vi "Measure.vi"(8 "error in (no error)":errorcluster, 11 "Instruments in":refnum<class "Instruments.lvclass">) -> (0 "error out":errorcluster, 3 "Instruments out":refnum<class "Instruments.lvclass">)   [LabVIEW 2023, in "Instruments.lvlib" / "Instruments.lvclass"]
doc: "<b>Measure</b>\nMust be overridden by descendent classes.\nCall parent method must be called <b>after</b> the override\n\n<b>Instrument </b> layer reads the measured private data, and enqueues the data for logging\n\nImmediate Descendants of the measure routine should override the measure routine by implementing class specific override methods. The immediate descendant is the only class that should override measure, and their descendants should provide an application speceific method for acquiring data. \n\nThis approach guarantees a common reporting method for instrument telemetry regardless of the specific device used."
uses:
  Library/Instruments.lvclass
  Library/Instruments.lvclass/Instruments.ctl
  builds/Framework/Engine.lvlibp/Engine/Accessors/Read Report Q.vi
  builds/Framework/Actor Framework.lvlibp/1abvi3w/vi.lib/ActorFramework/Actor/Read Actor Label.vi
  builds/Tools/QDMH.lvlibp/Private/Enqueue Single Element.vi
  builds/Tools/QDMH.lvlibp/Library/QDMH.lvclass
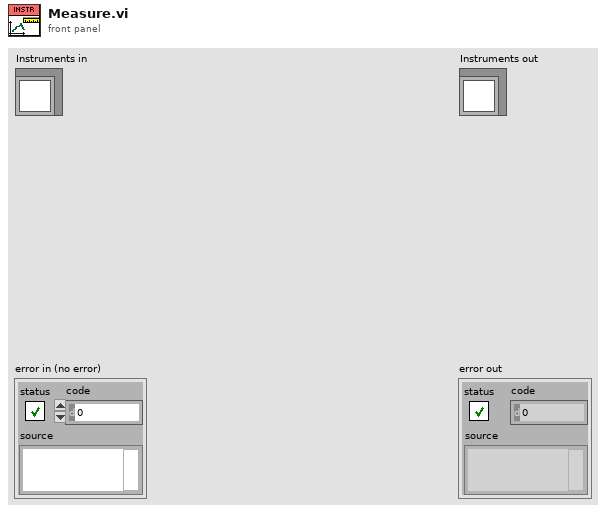
[diagram p1: front panel]
types:
  T1 = cluster{"Accessors:Actor Label":string, "Measured":waveform(dbl)[]}
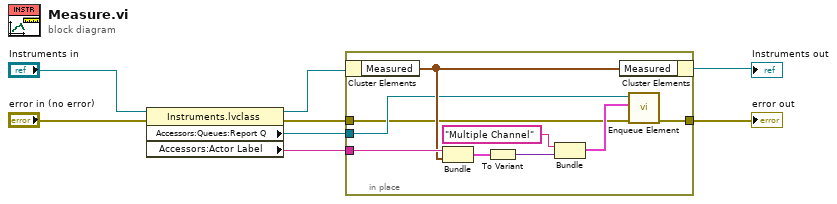
[diagram p0: block diagram]
diagram:
  n1 = property class="Instruments.lvclass"(reference="Instruments in", error in="error in (no error)") -> (reference out=w7:refnum<class "Instruments.lvclass">, error out=w4:errorcluster, "Accessors:Queues:Report Q"=w5:refnum<class "QDMH.lvclass">, "Accessors:Actor Label"=w1:string)
  n2 = in-place {
    in-place-border: w5 -> [w12]
    in-place-border: w4 -> [w10]
    in-place-border: [w9] -> w3
    in-place-border: w1 -> [w17]
    n3 = in-place-cluster #1(w7) -> ("Measured"=w16:waveform(dbl)[])
    n4 = Bundle("Accessors:Actor Label"=w17, "Measured"=w16) -> (w15:T1)  [unwired: 1 in]
    n5 = To Variant(anything=w15) -> (Variant=w14:variant)
    n6 = Bundle("Multiple Channel", "Variant"=w14) -> (w11:cluster{string, "Variant":variant})  [unwired: 1 in]
    n7 = in-place-cluster #1("Measured"=w16) -> (→"Instruments out":refnum<class "Instruments.lvclass">)
    n8 = call-poly "Enqueue Element.vi"("error in (no error)"=w10, "Message"=w11, "QDMH in"=w12) -> ("error out"=w9:errorcluster)  [unwired: 7 in, 1 out]
  }
  "error out" <- w3
